vi "TCP-IP Link.Core.vi"(4 "Status Element":T3={"Cmd"="TCP-IP", "Sub"="Status", "Data1"=variant, "Data2"=variant}, 5 "Options":T1={"Status Notify En"=TRUE, "Auto Connect"=TRUE, "Packet Format"=enum."First 2 Bytes is Length (U16)"}, 6 "Rcv Data Element":T3={"Cmd"="TCP-IP", "Sub"="Rcv", "Data1"=variant, "Data2"=variant}, 7 "StatusCtrlRef":refnum<vi>, 9 "Config":T4={"IP"="127.0.0.1", "Port"=8510, "Listener"=FALSE}, 10 "Q_RcvData":refnum<queue>, 11 "Control Q Name":string="TCP-IP_Link") -> ()   [LabVIEW 2024, in "EQMF.lvlib" / "TCP-IP.lvlib"]
uses:
  TCP-IP.lvlib
  Queues/Q.Element.ctl
  Controls/TCP-IP Link.Config.ctl
  Controls/TCP-IP Link.Options.ctl
  Controls/TCP-IP Link.Packet Format.ctl
  Controls/TCP-IP Link.Status.ctl
  Queues/Queue Utils.lvlib
panel:
  out "Close":bool
  out "connection ID":refnum<k5>
  out "Listener ID":refnum<k5>
  out "Exit":bool
  out "Connected":bool
  out "error out":errorcluster
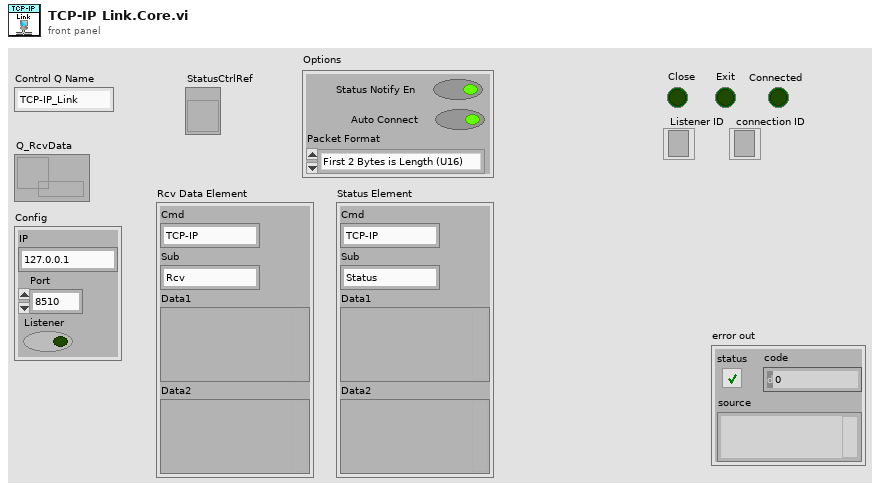
[diagram p1: front panel]
types:
  T1 = typedef "EQMF.lvlib/TCP-IP.lvlib/TCP-IP Link.Options.ctl" = cluster{"Status Notify En":bool, "Auto Connect":bool, "Packet Format":T2}
  T2 = typedef "EQMF.lvlib/TCP-IP.lvlib/TCP-IP Link.Packet Format.ctl" = enum16{"First 2 Bytes is Length (U16)", "First 3 Chars is Length"}
  T3 = typedef "EQMF.lvlib/Queue Utils.lvlib/Q.Element.ctl" = cluster{"Cmd":string, "Sub":string, "Data1":variant, "Data2":variant}
  T4 = typedef "EQMF.lvlib/TCP-IP.lvlib/TCP-IP Link.Config.ctl" = cluster{"IP":string, "Port":u16, "Listener":bool}
  T5 = typedef "EQMF.lvlib/TCP-IP.lvlib/TCP-IP Link.Status.ctl" = enum16{"Disconnected", "Connected", "Connecting", "Failed to Connect", "Listening"}
  T6 = cluster{"ConnectionID":refnum<k5>, "listenerID":refnum<k5>, "Connected":bool, "StatusCtrlRef":refnum<vi>, "CtrlRefEn":bool, "Options":T1, "Config":T4}
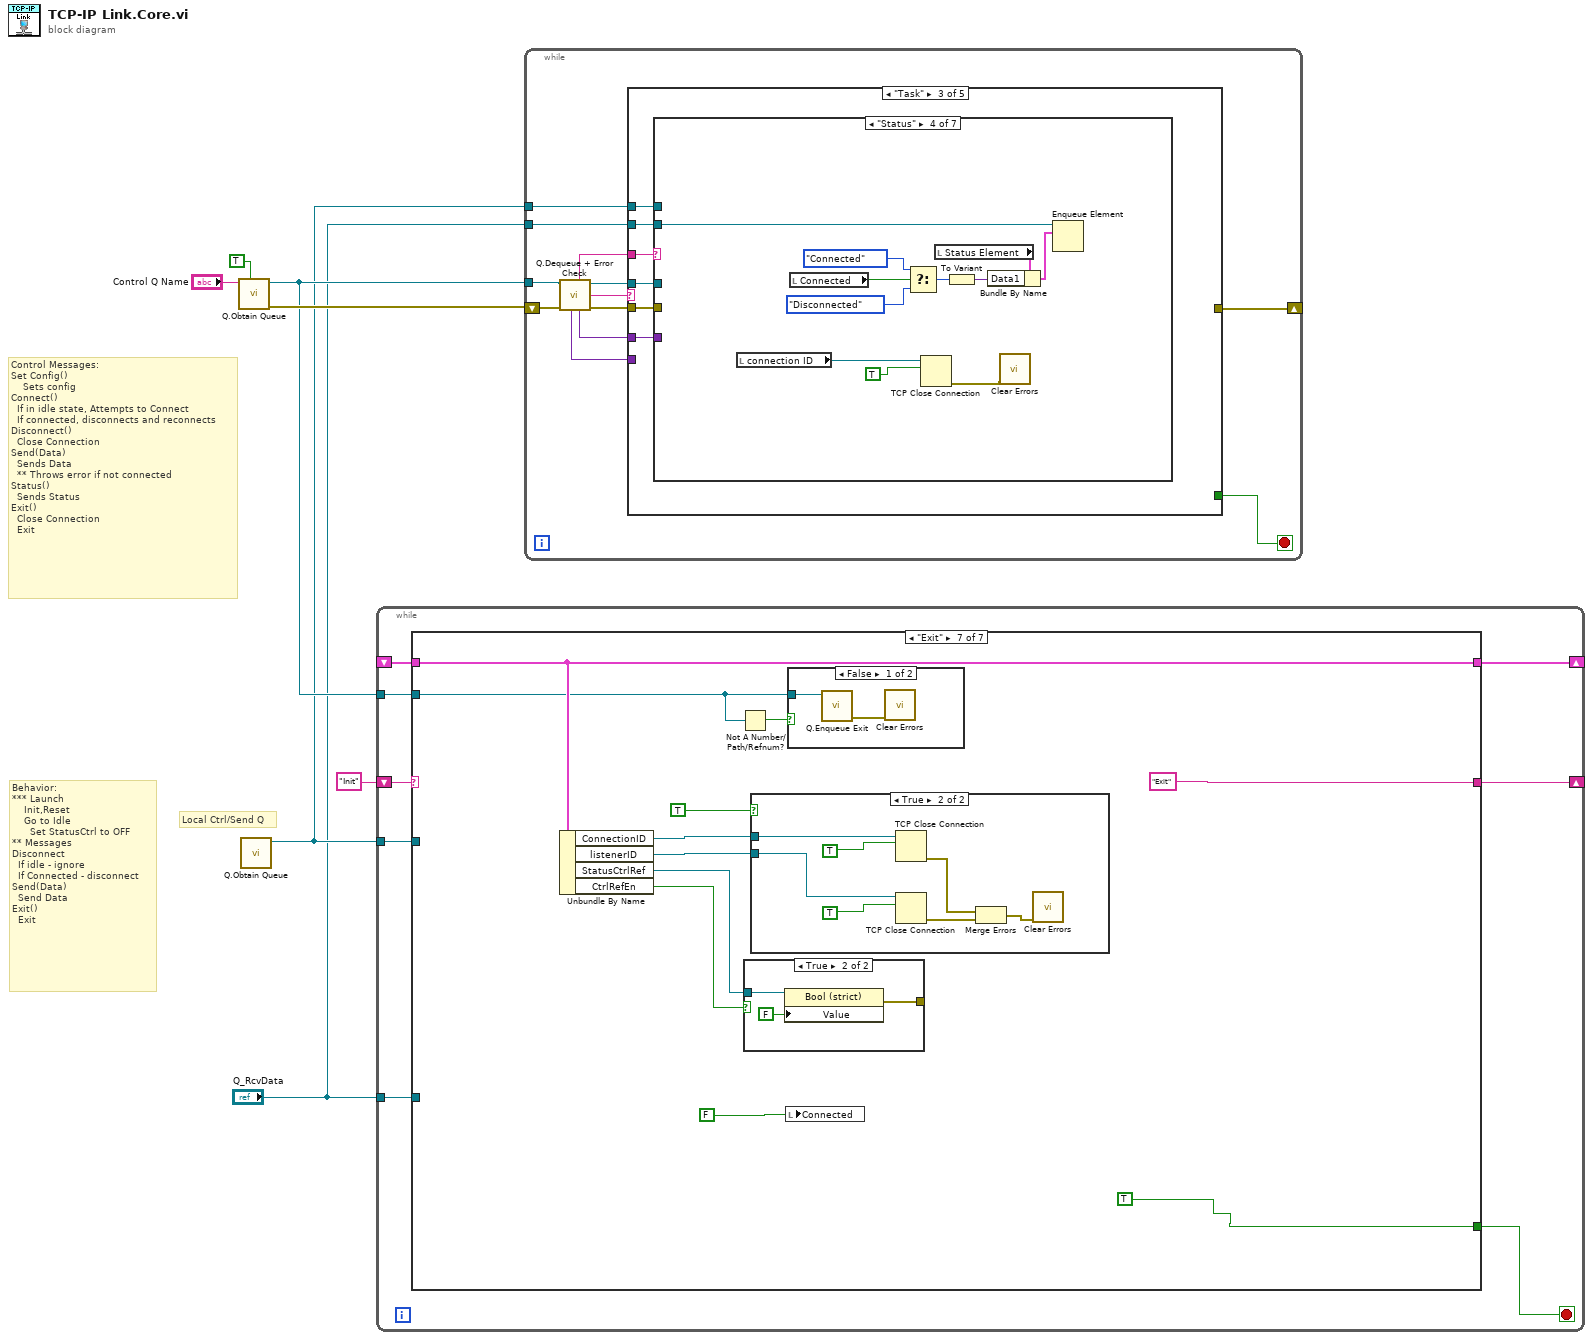
[diagram p0: block diagram]
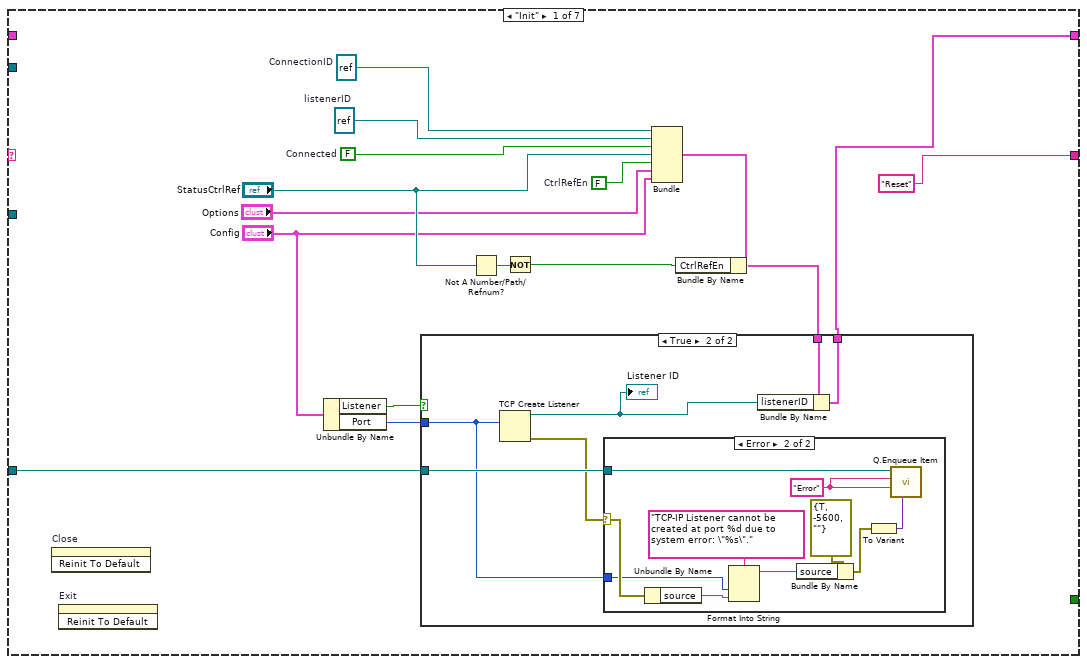
[diagram p2: hidden frame]
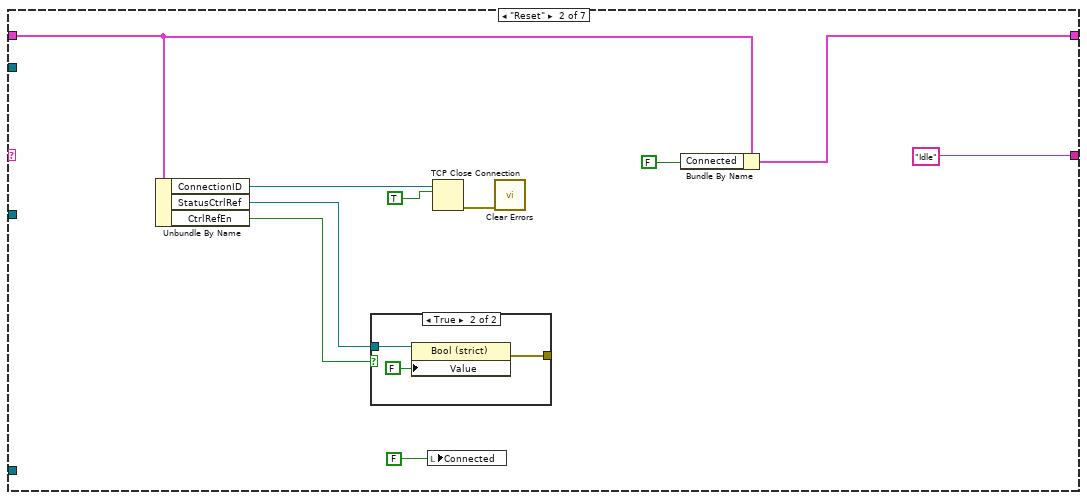
[diagram p5: hidden frame]
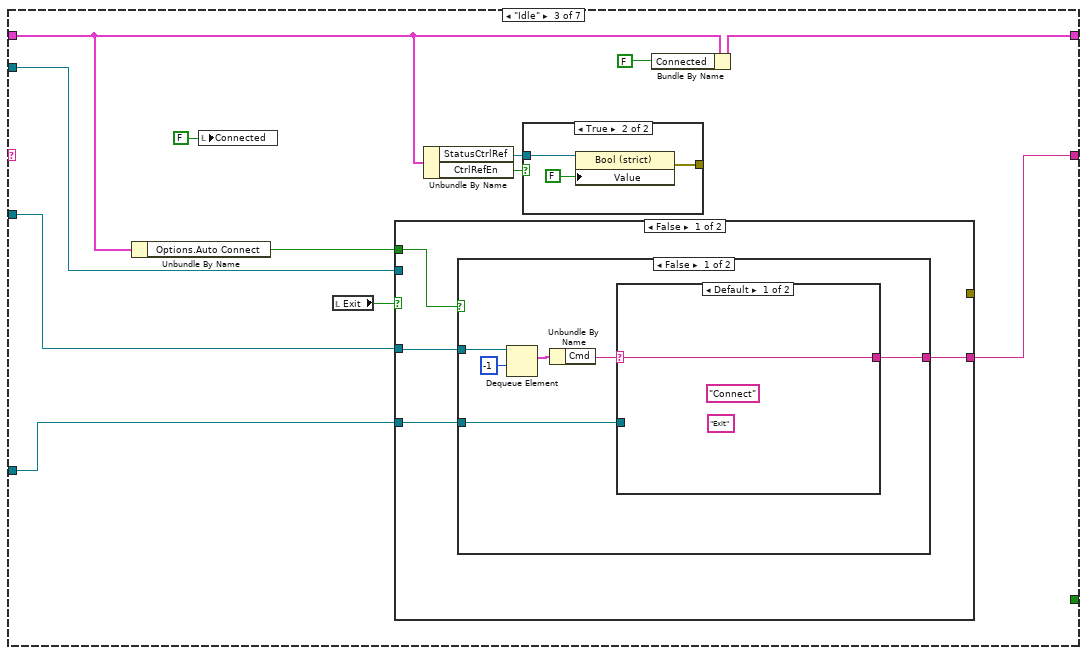
[diagram p7: hidden frame]
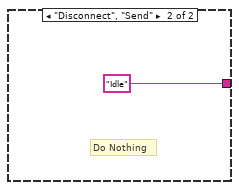
[diagram p9: hidden frame]
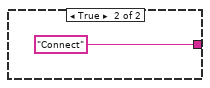
[diagram p10: hidden frame]
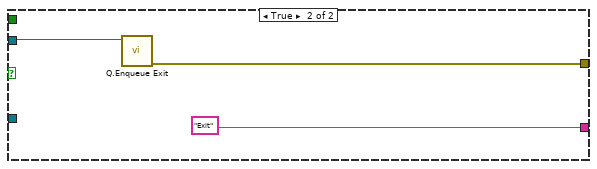
[diagram p11: hidden frame]
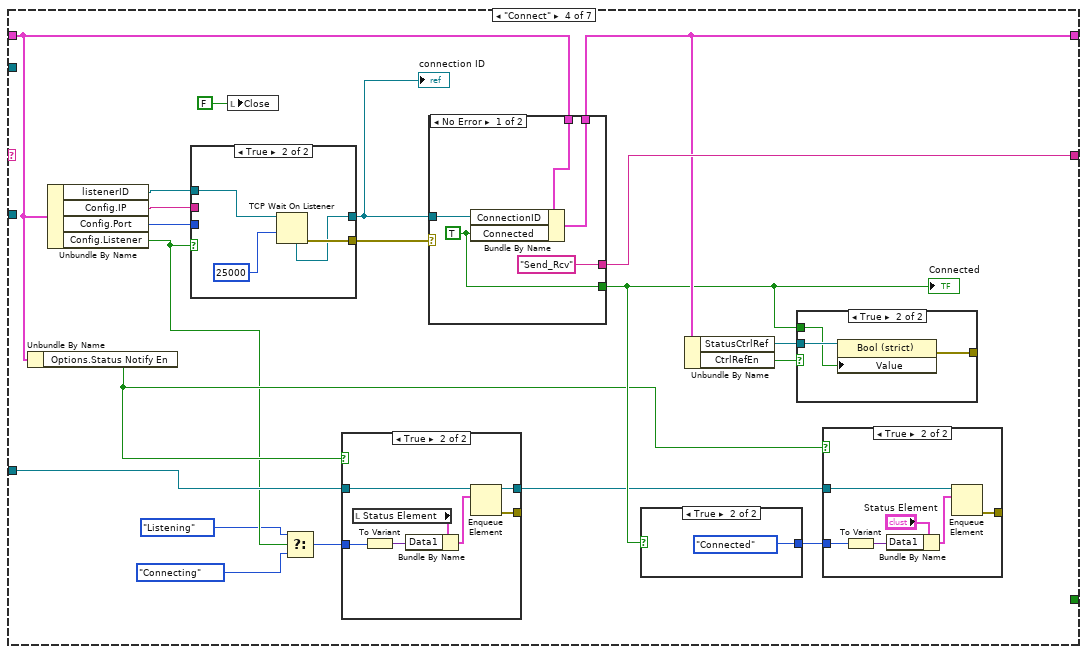
[diagram p12: hidden frame]
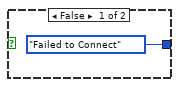
[diagram p14: hidden frame]
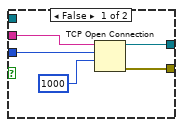
[diagram p17: hidden frame]
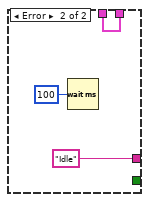
[diagram p18: hidden frame]
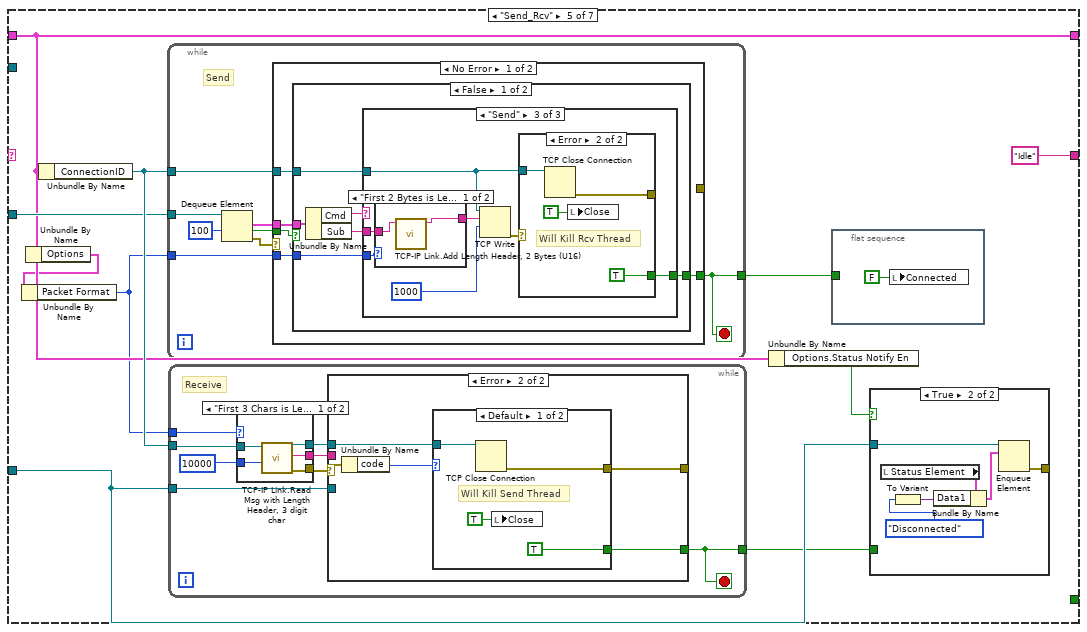
[diagram p19: hidden frame]
diagram:
  # "Local Ctrl/Send Q"
  # "Behavior:\n*** Launch\n    Init,Reset\n    Go to Idle\n      Set StatusCtrl to OFF\n** Messages\nDisconnect\n  If idle - ignore\n  If Connected - disconnect\nSend(Data)\n  Send Data\nExit()\n  Exit"
  # "Control Messages:\nSet Config()\n    Sets config\nConnect()\n  If in idle state, Attempts to Connect\n  If connected, disconnects and reconnects\nDisconnect()\n  Close Connection\nSend(Data)\n  Sends Data\n  ** Throws error if not connected\nStatus()\n  Sends Status \nExit()\n  Close Connection\n  Exit"
  n1 = call "Q.Obtain Queue.vi"("Enqueue Init"=TRUE, "Q Name"="Control Q Name") -> ("error out"=w6:errorcluster, "Q Out"=w4:refnum<queue>)  [unwired: 7 in, 1 out]
  n2 = call "Q.Obtain Queue.vi"() -> ("Q Out"=w2:refnum<queue>)  [unwired: 9 in, 2 out]
  n3 = while {
    shift-right: [w13] -> _
    shift-left: _ -> [w14]
    shift-right: [w9] -> _
    shift-left: "Init" -> [w15]
    tunnel: w2 -> [w11]
    tunnel: "Q_RcvData" -> [w10]
    tunnel: w4 -> [w8]
    stop <- w12 stop-if-true
    n4 = case shown="\"Exit\"" w15 {
      tunnel: w14 -> [_ w56 w63 w94 w151 w244 w252]
      tunnel: [w19 w55 w73 w103 w151 w244 w252] -> w13
      tunnel: ["Reset" "Idle" w71 w110 "Idle" "Reset" "Exit"] -> w9
      tunnel: [_ _ _ _ _ _ TRUE] -> w12
      tunnel: w11 -> [_ _ w66 _ w156 _ _]
      tunnel: w10 -> [w18 _ w65 w101 w155 _ _]
      tunnel: w8 -> [_ _ w69 _ _ _ w247]
      frame "Init" {
        w25 = FALSE  # CtrlRefEn
        w28 = FALSE  # Connected
        w29 = refnum<k5> refnum  # listenerID
        w30 = refnum<k5> refnum  # ConnectionID
        n5 = invoke on="Close" class="Bool (strict)" method="Reinit To Default"() -> ()  [unwired: 3 in, 3 out]
        n6 = invoke on="Exit" class="Bool (strict)" method="Reinit To Default"() -> ()  [unwired: 3 in, 3 out]
        n7 = Unbundle By Name("Config") -> ("Listener"=w21:bool, "Port"=w16:u16)
        n8 = Not A Number/Path/Refnum?(number/path/refnum="StatusCtrlRef") -> (NaN/Path/Refnum?=w26:bool)
        n9 = Not(x=w26) -> (.not. x?=w23:bool)
        n10 = Bundle("ConnectionID"=w30, "listenerID"=w29, "Connected"=w28, "StatusCtrlRef"="StatusCtrlRef", "CtrlRefEn"=w25, "Options"="Options", "Config"="Config") -> (w24:T6)  [unwired: 1 in]
        n11 = Bundle By Name(cluster=w24, "CtrlRefEn"=w23) -> (w20:T6)
        n12 = case shown="True" w21 {
          tunnel: w16 -> [_ w34]
          tunnel: w20 -> [w32 w38]
          tunnel: [w32 w37] -> w19
          tunnel: w18 -> [_ w36]
          frame False {
          }
          frame True {
            n13 = TCP Create Listener(10:w34) -> (0:w35:errorcluster, 3:w33:refnum<k5>)  [unwired: 4 in, 1 out]
            "Listener ID" <- w33
            n14 = case shown="Error" w35 {
              selector: w35 -> [_ w41]
              tunnel: w36 -> [_ w42]
              tunnel: w34 -> [_ w39]
              frame No Error {
              }
              frame Error {
                w43 = "Error" ("Cmd")
                n15 = Unbundle By Name(w41) -> ("source"=w40:string)
                n16 = Format Into String(format string="TCP-IP Listener cannot be created at port %d due to system error: \"%s\"." ("source"), w39, w40) -> (resulting string=w48:string)  [unwired: 2 in, 1 out]
                n17 = Bundle By Name(cluster=errorcluster {"status"=TRUE, "code"=-5600, "source"=""} ("error constant"), "source"=w48) -> (w47:errorcluster)
                n18 = To Variant(anything=w47) -> (Variant=w46:variant)
                n19 = call "Q.Enqueue Item.vi"("Data1"=w46, "Sub"=w43, "Cmd"=w43, "Q In"=w42) -> ()  [unwired: 6 in, 2 out]
              }
            }
            n20 = Bundle By Name(cluster=w38, "listenerID"=w33) -> (w37:T6)
          }
        }
      }
      frame "Reset" {
        n21 = Unbundle By Name(w56) -> ("ConnectionID"=w58:refnum<k5>, "StatusCtrlRef"=w52:refnum<vi>, "CtrlRefEn"=w51:bool)
        n22 = case shown="True" w51 {
          tunnel: w52 -> [_ w61]
          tunnel: [_ w59] -> _
          frame False {
          }
          frame True {
            n23 = property class="Bool (strict)"(reference=w61, "Value"=FALSE) -> (error out=w59:errorcluster)  [unwired: 1 in, 1 out]
          }
        }
        n24 = local write "Connected"(FALSE ("Value")) -> ()
        n25 = TCP Close Connection(connection ID=w58, abort (F)=TRUE) -> (error out=w49:errorcluster)  [unwired: 1 in, 1 out]
        n26 = call <vilib>:"Clear Errors.vi"("error in (no error)"=w49) -> ()  [unwired: 5 in, 2 out]
        n27 = Bundle By Name(cluster=w56, "Connected"=FALSE) -> (w55:T6)
      }
      frame "Idle" {
        n28 = Unbundle By Name(w63) -> ("Options.Auto Connect"=w62:bool)
        n29 = local write "Connected"(FALSE ("Connected")) -> ()
        n30 = local read "Exit"() -> (w70:bool)
        n31 = case shown="False" w70 {
          tunnel: [w79 "Exit"] -> w71
          tunnel: w69 -> [_ w91]
          tunnel: [_ w90] -> _
          tunnel: w66 -> [w80 _]
          tunnel: w65 -> [w78 _]
          tunnel: w62 -> [w77 _]
          frame False {
            n32 = case shown="False" w77 {
              tunnel: w80 -> [w86 _]
              tunnel: [w82 "Connect"] -> w79
              tunnel: w78 -> [w81 _]
              frame False {
                n33 = Dequeue Element(queue=w86, timeout in ms (-1)=-1) -> (element=w85:T3)  [unwired: 1 in, 3 out]
                n34 = Unbundle By Name(w85) -> ("Cmd"=w83:string)
                n35 = case shown="Default" w83 {
                  selector: w83 -> [w87 _]
                  tunnel: [w87 "Idle"] -> w82
                  tunnel: w81 -> [_ _]
                  frame Default {
                    (unwired) "Exit"
                    (unwired) "Connect"
                  }
                  frame "Disconnect", "Send" {
                    # "Do Nothing"
                  }
                }
              }
              frame True {
              }
            }
          }
          frame True {
            n36 = call "Q.Enqueue Exit.vi"("Q In"=w91) -> ("error out"=w90:errorcluster)  [unwired: 9 in, 1 out]
          }
        }
        n37 = Unbundle By Name(w63) -> ("StatusCtrlRef"=w68:refnum<vi>, "CtrlRefEn"=w67:bool)
        n38 = case shown="True" w67 {
          tunnel: w68 -> [_ w76]
          tunnel: [_ w75] -> _
          frame False {
          }
          frame True {
            n39 = property class="Bool (strict)"(reference=w76, "Value"=FALSE ("Connected")) -> (error out=w75:errorcluster)  [unwired: 1 in, 1 out]
          }
        }
        n40 = Bundle By Name(cluster=w63, "Connected"=FALSE) -> (w73:T6)
      }
      frame "Connect" {
        n41 = Unbundle By Name(w94) -> ("Options.Status Notify En"=w99:bool)
        n42 = Unbundle By Name(w94) -> ("listenerID"=w93:refnum<k5>, "Config.IP"=w112:string, "Config.Port"=w111:u16, "Config.Listener"=w98:bool)
        n43 = case shown="True" w98 {
          tunnel: w112 -> [w136 _]
          tunnel: w111 -> [w135 _]
          tunnel: [w133 w139] -> w108
          tunnel: [w132 w140] -> w109
          tunnel: w93 -> [_ w137]
          frame False {
            n44 = TCP Open Connection(address=w136, remote port or service name=w135, timeout ms (60000)=1000) -> (connection ID=w133:refnum<k5>, error out=w132:errorcluster)  [unwired: 2 in]
          }
          frame True {
            n45 = TCP Wait On Listener(9:25000 ("timeout ms (wait forever: -1)"), 11:w137) -> (0:w140:errorcluster, 4:w139:refnum<k5>)  [unwired: 2 in, 3 out]
          }
        }
        "connection ID" <- w108
        n46 = local write "Close"(FALSE ("Reset")) -> ()
        n47 = Select(t=TCP-IP_Link.Status."Listening", s=w98, f=TCP-IP_Link.Status."Connecting") -> (s? t:f=w95:T5)
        n48 = case shown="True" w99 {
          tunnel: w101 -> [w113 w118]
          tunnel: [_ w116] -> _
          tunnel: [w113 w115] -> w100
          tunnel: w95 -> [_ w114]
          frame False {
          }
          frame True {
            n49 = local read "Status Element"() -> (w117:T3)
            n50 = To Variant(anything=w114) -> (Variant=w119:variant)
            n51 = Bundle By Name(cluster=w117, "Data1"=w119) -> (w120:T3)
            n52 = Enqueue Element(queue=w118, element=w120) -> (queue out=w115:refnum<queue>, error out=w116:errorcluster)  [unwired: 2 in, 1 out]
          }
        }
        n53 = case shown="No Error" w109 {
          tunnel: w94 -> [w145 w146]
          tunnel: w108 -> [w144 _]
          tunnel: [w143 w146] -> w103
          tunnel: ["Send_Rcv" "Idle"] -> w110
          tunnel: [w141 _] -> w102
          frame No Error {
            w141 = TRUE ("Connected")
            n54 = Bundle By Name(cluster=w145, "ConnectionID"=w144, "Connected"=w141) -> (w143:T6)
          }
          frame Error {
            n55 = Wait (ms)(milliseconds to wait=u32 100) -> ()  [unwired: 1 out]
          }
        }
        "Connected" <- w102
        n56 = case shown="True" w102 {
          tunnel: [TCP-IP_Link.Status."Failed to Connect" TCP-IP_Link.Status."Connected"] -> w104
          frame False {
          }
          frame True {
          }
        }
        n57 = Unbundle By Name(w103) -> ("StatusCtrlRef"=w106:refnum<vi>, "CtrlRefEn"=w105:bool)
        n58 = case shown="True" w105 {
          tunnel: w106 -> [_ w131]
          tunnel: [_ w130] -> _
          tunnel: w102 -> [_ w129]
          frame False {
          }
          frame True {
            n59 = property class="Bool (strict)"(reference=w131, "Value"=w129) -> (error out=w130:errorcluster)  [unwired: 1 in, 1 out]
          }
        }
        n60 = case shown="True" w99 {
          tunnel: w104 -> [_ w125]
          tunnel: w100 -> [_ w124]
          tunnel: [_ w123] -> _
          frame False {
          }
          frame True {
            n61 = To Variant(anything=w125) -> (Variant=w126:variant)
            n62 = Bundle By Name(cluster="Status Element", "Data1"=w126) -> (w128:T3)
            n63 = Enqueue Element(queue=w124, element=w128) -> (error out=w123:errorcluster)  [unwired: 2 in, 2 out]
          }
        }
      }
      frame "Send_Rcv" {
        n64 = Unbundle By Name(w151) -> ("Options"=w150:T1)
        n65 = Unbundle By Name(w150) -> ("Packet Format"=w149:T2)
        n66 = Unbundle By Name(w151) -> ("ConnectionID"=w158:refnum<k5>)
        n67 = while {
          tunnel: w156 -> [w206]
          tunnel: w158 -> [w204]
          tunnel: [w200] -> w153
          tunnel: w149 -> [w199]
          stop <- w200 stop-if-true
          # "Send"
          n68 = Dequeue Element(queue=w206, timeout in ms (-1)=100) -> (element=w202:T3, timed out?=w203:bool, error out=w201:errorcluster)  [unwired: 1 in, 1 out]
          n69 = case shown="No Error" w201 {
            tunnel: [w211 TRUE] -> w200
            tunnel: w204 -> [w210 w239]
            tunnel: w203 -> [w209 _]
            tunnel: w202 -> [w208 _]
            tunnel: [_ w238] -> _
            tunnel: w199 -> [w207 _]
            frame No Error {
              n70 = case shown="False" w209 {
                tunnel: [w217 w236] -> w211
                tunnel: w208 -> [w214 _]
                tunnel: w210 -> [w216 _]
                tunnel: w207 -> [w212 _]
                frame False {
                  n71 = Unbundle By Name(w214) -> ("Cmd"=w213:string, "Sub"=w215:string)
                  n72 = case shown="\"Send\"" w213 {
                    tunnel: [_ w219 w227] -> w217
                    tunnel: w216 -> [_ w220 w226]
                    tunnel: w215 -> [_ _ w222]
                    tunnel: w212 -> [_ _ w221]
                    frame Default {
                    }
                    frame "Disconnect", "Exit" {
                      w219 = TRUE ("Close")
                      n73 = TCP Close Connection(connection ID=w220) -> (error out=w218:errorcluster)  [unwired: 2 in, 1 out]
                      n74 = local write "Close"(w219) -> ()
                      n75 = call <vilib>:"Clear Errors.vi"("error in (no error)"=w218) -> ()  [unwired: 5 in, 2 out]
                    }
                    frame "Send" {
                      n76 = case shown="\"First 2 Bytes is Length (U16)\", Default" w221 {
                        tunnel: [w229 w231] -> w224
                        tunnel: w222 -> [w228 w230]
                        frame "First 2 Bytes is Length (U16)", Default {
                          n77 = call "TCP-IP Link.Add Length Header, 2 Bytes (U16).vi"("Message"=w228) -> ("Message + Header"=w229:string)  [unwired: 10 in]
                        }
                        frame "First 3 Chars is Length" {
                          n78 = call "TCP-IP Link.Add Length Header, 3 Chars.vi"("Message"=w230) -> ("Message + Header"=w231:string)  [unwired: 10 in]
                        }
                      }
                      n79 = TCP Write(connection ID=w226, data in=w224, 9:1000 ("timeout ms (25000)")) -> (error out=w225:errorcluster)  [unwired: 1 in, 2 out]
                      n80 = case shown="Error" w225 {
                        tunnel: w226 -> [_ w234]
                        tunnel: [_ TRUE] -> w227
                        tunnel: [_ w233] -> _
                        frame No Error {
                        }
                        frame Error {
                          # "Will Kill Rcv Thread"
                          n81 = TCP Close Connection(connection ID=w234) -> (error out=w233:errorcluster)  [unwired: 2 in, 1 out]
                          n82 = local write "Close"(TRUE ("Close")) -> ()
                        }
                      }
                    }
                  }
                }
                frame True {
                  # "This time out allows ability to stop/exit"
                  # "Do nothing\nTimed Out"
                  n83 = local read "Close"() -> (w236:bool)
                }
              }
            }
            frame Error {
              # "Exit"
              # "Will Kill Rcv Thread"
              n84 = TCP Close Connection(connection ID=w239) -> (error out=w238:errorcluster)  [unwired: 2 in, 1 out]
              n85 = local write "Exit"(TRUE ("Close")) -> ()
              n86 = local write "Close"(TRUE ("Close")) -> ()
            }
          }
        }
        n87 = while {
          tunnel: w155 -> [w173]
          tunnel: w158 -> [w171]
          tunnel: [w168] -> w154
          tunnel: w149 -> [w166]
          stop <- w168 stop-if-true
          # "Receive"
          n88 = case shown="\"First 3 Chars is Length\"" w166 {
            tunnel: [w178 w183] -> w172
            tunnel: w171 -> [w177 w182]
            tunnel: [w176 w181] -> w170
            tunnel: [w175 w180] -> w169
            tunnel: 10000 ("timeout ms (25000)") -> [w174 w179]
            frame "First 3 Chars is Length" {
              n89 = call "TCP-IP Link.Read Msg with Length Header, 3 digit char.vi"("Timeoutms"=w174, "ConID"=w177) -> ("Error Out"=w175:errorcluster, "data out"=w176:string, "ConID Out"=w178:refnum<k5>)  [unwired: 6 in, 1 out]
            }
            frame "First 2 Bytes is Length (U16)" {
              n90 = call "TCP-IP Link.Read Msg with Length Header, 2 Byte U16.vi"("Timeoutms"=w179, "ConID"=w182) -> ("Error Out"=w180:errorcluster, "data out"=w181:string, "ConID Out"=w183:refnum<k5>)  [unwired: 6 in, 1 out]
            }
          }
          n91 = case shown="Error" w169 {
            selector: w169 -> [_ w191]
            tunnel: w173 -> [w186 _]
            tunnel: w172 -> [_ w193]
            tunnel: [_ w194] -> w168
            tunnel: [w184 w192] -> _
            tunnel: w170 -> [w188 _]
            frame No Error {
              n92 = To Variant(anything=w188) -> (Variant=w187:variant)
              n93 = Bundle By Name(cluster="Rcv Data Element", "Data1"=w187) -> (w185:T3)
              n94 = Enqueue Element(queue=w186, element=w185) -> (error out=w184:errorcluster)  [unwired: 2 in, 2 out]
            }
            frame Error {
              n95 = Unbundle By Name(w191) -> ("code"=w190:i32)
              n96 = case shown="Default" w190 {
                tunnel: [TRUE _] -> w194
                tunnel: w193 -> [w197 _]
                tunnel: [w196 _] -> w192
                frame Default {
                  # "Will Kill Send Thread"
                  n97 = TCP Close Connection(connection ID=w197) -> (error out=w196:errorcluster)  [unwired: 2 in, 1 out]
                  n98 = local write "Close"(TRUE ("Close")) -> ()
                }
                frame 56 {
                  (unwired) 56 items=["No Error", "Argument Error", "Memory Full", "Out of Zone", "End of File", "File Already Open", "Generic File IO Error", "File Not Found", "File Permission Error", "Disk Full", "Duplicate Path", "Too Many Files Open", "Not Enabled", "Resource File Not Found", "Cannot Add Resource", "Resource Not Found", "Image Not Found", "Image Memory Error", "Pen Does Not Exist", "Config Bad Type", "Config Token Not Found", "Config Parse Error", "Config Memory Error", "Bad External Code Format", "Bad External Code Offset", "External Code Not Present", "Null Window", "Destroy Window Mixup", "Null Menu", "Print Aborted", "Bad Print Record", "Print Driver Error", "Windows Error During Print", "Memory Error During Print", "Print Dialog Error", "Generic Print Error", "Invalid Device Refnum", "Device Not Found", "Device Parameter Error", "Device Unit Error", "Can't Open Device", "Device Call Aborted", "Generic Error", "Cancelled By User", "Object ID Too Low", "Object ID Too High", "Object Not In Heap", "Unknown Heap", "Bad DefProc ID", "DefProc Not In Table", "Message Out Of Range", "Null Method", "Unknown Message", "Manager Call Not Supported", "Bad address", "Connection In progress", "Connection timed out", "Connection is already in progress", "Network attribute not supported", "Network error", "Address in use", "System out of memory", "Connection aborted", "Connection refused", "Connection is not connected", "Connection is already connected", "Connection closed", "Initialize error (interapplication manager)", "Bad occurrence", "Wait on unbound occurrence handler", "Occurrence queue overflow", "Bad path", "Semaphore not signaled", "Unrecognized type (interapplication manager)"] ("2nd Error to Convert")
                  # "Do Nothing"
                }
              }
            }
          }
        }
        n99 = Unbundle By Name(w151) -> ("Options.Status Notify En"=w152:bool)
        n100 = flat-sequence {
          tunnel: w153 -> [_]
          frame #0 {
            n101 = local write "Connected"(FALSE ("Connected")) -> ()
          }
        }
        n102 = case shown="True" w152 {
          tunnel: w155 -> [_ w163]
          tunnel: [_ w160] -> _
          tunnel: w154 -> [_ _]
          frame False {
          }
          frame True {
            n103 = local read "Status Element"() -> (w162:T3)
            n104 = To Variant(anything=TCP-IP_Link.Status."Disconnected") -> (Variant=w164:variant)
            n105 = Bundle By Name(cluster=w162, "Data1"=w164) -> (w165:T3)
            n106 = Enqueue Element(queue=w163, element=w165) -> (error out=w160:errorcluster)  [unwired: 2 in, 2 out]
          }
        }
      }
      frame "Error", Default {
        n107 = Wait (ms)(milliseconds to wait=u32 100) -> ()  [unwired: 1 out]
      }
      frame "Exit" {
        n108 = Unbundle By Name(w252) -> ("ConnectionID"=w254:refnum<k5>, "listenerID"=w253:refnum<k5>, "StatusCtrlRef"=w250:refnum<vi>, "CtrlRefEn"=w249:bool)
        n109 = Not A Number/Path/Refnum?(number/path/refnum=w247) -> (NaN/Path/Refnum?=w246:bool)
        n110 = case shown="True" w249 {
          tunnel: w250 -> [_ w267]
          tunnel: [_ w265] -> _
          frame False {
          }
          frame True {
            n111 = property class="Bool (strict)"(reference=w267, "Value"=FALSE) -> (error out=w265:errorcluster)  [unwired: 1 in, 1 out]
          }
        }
        n112 = case shown="True" TRUE {
          tunnel: w254 -> [_ w262]
          tunnel: w253 -> [_ w259]
          frame False {
          }
          frame True {
            n113 = TCP Close Connection(connection ID=w262, abort (F)=TRUE) -> (error out=w257:errorcluster)  [unwired: 1 in, 1 out]
            n114 = TCP Close Connection(connection ID=w259, abort (F)=TRUE) -> (error out=w258:errorcluster)  [unwired: 1 in, 1 out]
            n115 = Merge Errors(w257, w258) -> (w256:errorcluster)
            n116 = call <vilib>:"Clear Errors.vi"("error in (no error)"=w256) -> ()  [unwired: 5 in, 2 out]
          }
        }
        n117 = local write "Connected"(FALSE ("Value")) -> ()
        n118 = case shown="False" w246 {
          tunnel: w247 -> [w263 _]
          frame False {
            n119 = call "Q.Enqueue Exit.vi"("Q In"=w263) -> ("error out"=w264:errorcluster)  [unwired: 9 in, 1 out]
            n120 = call <vilib>:"Clear Errors.vi"("error in (no error)"=w264) -> ()  [unwired: 5 in, 2 out]
          }
          frame True {
          }
        }
      }
    }
  }
  n121 = while {
    tunnel: w4 -> [w279]
    shift-right: [w271] -> _
    shift-left: w6 -> [w278]
    tunnel: w2 -> [w269]
    tunnel: "Q_RcvData" -> [w268]
    stop <- w270 stop-if-true
    n122 = call "Q.Dequeue + Error Check.vi"("Error In"=w278, "Q In"=w279) -> ("error out"=w275:errorcluster, "Cmd"=w277:string, "Q Out"=w276:refnum<queue>, "Data1"=w274:variant, "Sub"=w272:string, "Data2"=w273:variant)  [unwired: 4 in]
    n123 = case shown="\"Task\"" w277 {
      tunnel: w276 -> [_ _ w286 _ w346]
      tunnel: w275 -> [_ _ w287 w339 _]
      tunnel: w274 -> [_ _ w288 w337 _]
      tunnel: w273 -> [_ _ _ _ _]
      tunnel: w272 -> [_ _ w289 w340 _]
      tunnel: [_ _ _ errorcluster {"status"=FALSE, "code"=0, "source"=""} ("error constant") _] -> w271
      tunnel: [_ _ _ _ TRUE] -> w270
      tunnel: w269 -> [_ _ w285 _ w345]
      tunnel: w268 -> [_ _ w284 _ _]
      frame "Init" {
        n124 = invoke on="Exit" class="Bool (strict)" method="Reinit To Default"() -> ()  [unwired: 3 in, 3 out]
      }
      frame "Reset" {
        n125 = local read "connection ID"() -> (w282:refnum<k5>)
        n126 = TCP Close Connection(connection ID=w282, abort (F)=TRUE) -> (error out=w280:errorcluster)  [unwired: 1 in, 1 out]
        n127 = call <vilib>:"Clear Errors.vi"("error in (no error)"=w280) -> ()  [unwired: 5 in, 2 out]
        "Close" <- TRUE ("Reset")
      }
      frame "Task" {
        n128 = case shown="\"Status\"" w289 {
          tunnel: w288 -> [_ w292 _ _ _ w318 _]
          tunnel: w287 -> [_ _ _ _ _ _ _]
          tunnel: w286 -> [_ _ _ _ w313 _ w335]
          tunnel: w285 -> [_ _ w297 _ _ w319 _]
          tunnel: w284 -> [_ _ _ w307 _ w315 _]
          frame Default {
          }
          frame "Set Config" {
            n129 = Variant To Data(type=T4 {"IP"="127.0.0.1", "Port"=8500, "Listener"=FALSE} ("Config"), Variant=w292) -> (data=w291:T4)  [unwired: 1 in, 1 out]
            n130 = local write "Config"(w291) -> ()
          }
          frame "Connect" {
            n131 = local read "connection ID"() -> (w295:refnum<k5>)
            n132 = call "Q.Enqueue Item.vi"("Cmd"="Disconnect", "Q In"=w297) -> ("Q Out"=w298:refnum<queue>)  [unwired: 8 in, 1 out]
            n133 = TCP Close Connection(connection ID=w295, abort (F)=TRUE) -> (error out=w294:errorcluster)  [unwired: 1 in, 1 out]
            n134 = call "Q.Enqueue Item.vi"("Cmd"="Connect", "Q In"=w298) -> ()  [unwired: 8 in, 2 out]
            n135 = call <vilib>:"Clear Errors.vi"("error in (no error)"=w294) -> ()  [unwired: 5 in, 2 out]
          }
          frame "Status" {
            n136 = local read "connection ID"() -> (w302:refnum<k5>)
            n137 = local read "Connected"() -> (w303:bool)
            n138 = Select(t=TCP-IP_Link.Status."Connected", s=w303, f=TCP-IP_Link.Status."Disconnected") -> (s? t:f=w306:T5)
            n139 = TCP Close Connection(connection ID=w302, abort (F)=TRUE) -> (error out=w301:errorcluster)  [unwired: 1 in, 1 out]
            n140 = local read "Status Element"() -> (w308:T3)
            n141 = To Variant(anything=w306) -> (Variant=w309:variant)
            n142 = Bundle By Name(cluster=w308, "Data1"=w309) -> (w310:T3)
            n143 = call <vilib>:"Clear Errors.vi"("error in (no error)"=w301) -> ()  [unwired: 5 in, 2 out]
            n144 = Enqueue Element(queue=w307, element=w310) -> ()  [unwired: 2 in, 3 out]
          }
          frame "Disconnect" {
            n145 = call "Q.Enqueue Reset.vi"("Top of Q(T)"=FALSE, "Flush Queue(T)"=FALSE, "Q In"=w313) -> ()  [unwired: 7 in, 2 out]
          }
          frame "Send" {
            n146 = Variant To Data(type="", Variant=w318) -> (data=w316:string)  [unwired: 1 in, 1 out]
            n147 = local read "Connected"() -> (w314:bool)
            n148 = case shown="True" w314 {
              tunnel: w319 -> [_ w327]
              tunnel: w316 -> [_ w325]
              tunnel: w315 -> [w321 _]
              tunnel: [w320 _] -> _
              frame False {
                w324 = "Error" ("Cmd")
                n149 = To Variant(anything=errorcluster {"status"=TRUE, "code"=-5600, "source"="TCP-IP link not connected, Cannot execute Send command."} ("error constant")) -> (Variant=w323:variant)
                n150 = call "Q.Enqueue Item.vi"("Data1"=w323, "Sub"=w324, "Cmd"=w324, "Q In"=w321) -> ("error out"=w320:errorcluster)  [unwired: 6 in, 1 out]
              }
              frame True {
                n151 = call "Q.Enqueue Item.vi"("Sub"=w325, "Cmd"="Send", "Q In"=w327) -> ()  [unwired: 7 in, 2 out]
              }
            }
          }
          frame "Exit" {
            n152 = call "Q.Enqueue Exit.vi"("Q In"=w335) -> ()  [unwired: 9 in, 2 out]
            n153 = local read "connection ID"() -> (w331:refnum<k5>)
            n154 = local read "Listener ID"() -> (w330:refnum<k5>)
            n155 = TCP Close Connection(connection ID=w331, abort (F)=TRUE) -> (error out=w333:errorcluster)  [unwired: 1 in, 1 out]
            n156 = TCP Close Connection(connection ID=w330, abort (F)=TRUE) -> (error out=w332:errorcluster)  [unwired: 1 in, 1 out]
            n157 = Merge Errors(w333, w332) -> (w334:errorcluster)
            n158 = call <vilib>:"Clear Errors.vi"("error in (no error)"=w334) -> ()  [unwired: 5 in, 2 out]
          }
        }
      }
      frame "Error", Default {
        n159 = case shown="\"Clear\", Default" w340 {
          tunnel: w339 -> [_ w344]
          tunnel: [w342 w344] -> w338
          tunnel: w337 -> [w341 _]
          frame "Error" {
            n160 = Variant To Data(type=errorcluster {"status"=FALSE, "code"=0, "source"=""} ("error constant"), Variant=w341) -> (data=w342:errorcluster)  [unwired: 1 in, 1 out]
          }
          frame "Clear", Default {
          }
        }
        "error out" <- w338
      }
      frame "Exit" {
        n161 = stacked-sequence {
          tunnel: w346 -> [_ _ w359]
          tunnel: w345 -> [_ _ w358]
          frame #0 {
            n162 = local write "Close"(TRUE ("Reset")) -> ()
            "Exit" <- TRUE ("Exit")
          }
          frame #1 {
            n163 = local read "connection ID"() -> (w351:refnum<k5>)
            n164 = local read "Listener ID"() -> (w350:refnum<k5>)
            n165 = TCP Close Connection(connection ID=w351, abort (F)=TRUE) -> (error out=w355:errorcluster)  [unwired: 1 in, 1 out]
            n166 = TCP Close Connection(connection ID=w350, abort (F)=TRUE) -> (error out=w354:errorcluster)  [unwired: 1 in, 1 out]
            n167 = Merge Errors(w355, w354) -> (w356:errorcluster)
            n168 = call <vilib>:"Clear Errors.vi"("error in (no error)"=w356) -> ()  [unwired: 5 in, 2 out]
          }
          frame #2 {
            n169 = Release Queue(queue=w359) -> ()  [unwired: 2 in, 3 out]
            n170 = call "Q.Enqueue Exit.vi"("Q In"=w358) -> ("error out"=w357:errorcluster)  [unwired: 9 in, 1 out]
            n171 = call <vilib>:"Clear Errors.vi"("error in (no error)"=w357) -> ()  [unwired: 5 in, 2 out]
          }
        }
      }
    }
  }
